vi "zad5.vi"() -> ()   [LabVIEW 2017]
panel:
  in  "Wybór podpunktu":enum32{"A", "B"}(radio)
  out "Suma":dbl
  in  "n":u64
  in  "r":dbl
  out "a(n)":dbl[](graph)
  in  "Wybierz ciąg":enum32{"Arytmetyczny", "Geometryczny"}(radio)
  in  "a1":dbl
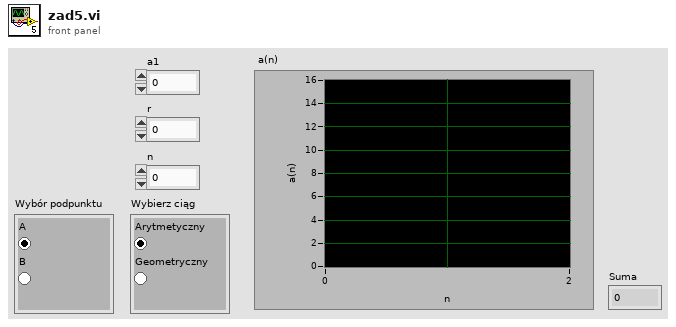
[diagram p1: front panel]
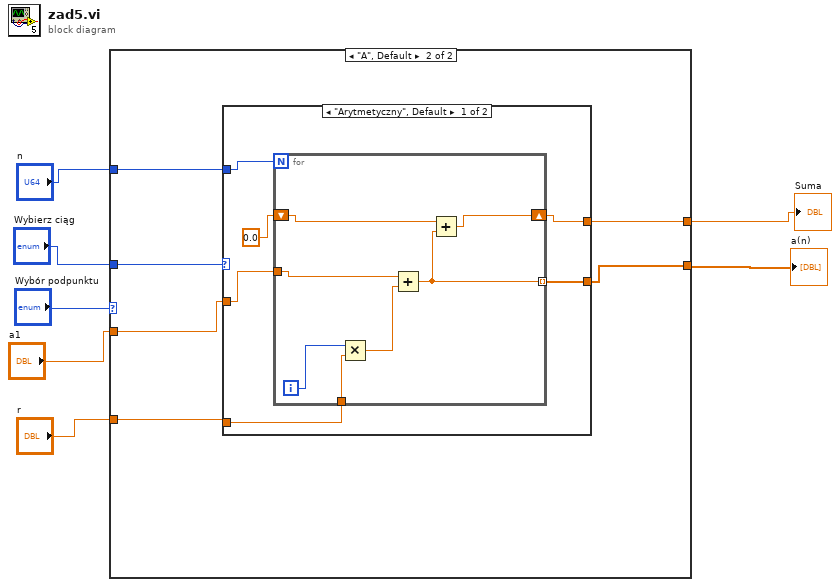
[diagram p0: block diagram]
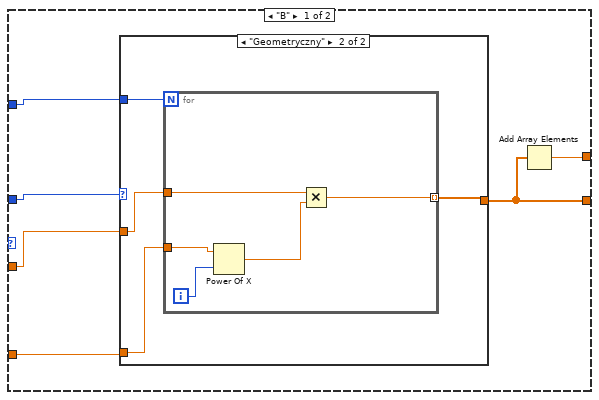
[diagram p2: hidden frame]
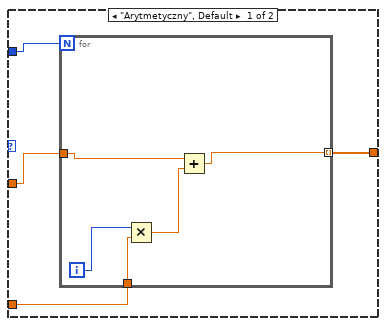
[diagram p3: hidden frame]
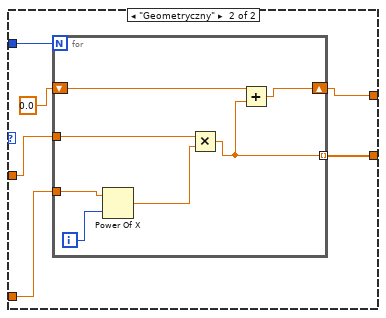
[diagram p4: hidden frame]
diagram:
  n1 = case shown="\"A\", Default" "Wybór podpunktu" {
    tunnel: [w8 w37] -> w2
    tunnel: "n" -> [w13 w36]
    tunnel: "r" -> [w10 w35]
    tunnel: "Wybierz ciąg" -> [w12 w34]
    tunnel: "a1" -> [w11 w33]
    tunnel: [w9 w32] -> w1
    frame "B" {
      n2 = case shown="\"Geometryczny\"" w12 {
        tunnel: w11 -> [w17 w25]
        tunnel: w10 -> [w16 w26]
        tunnel: w13 -> [w15 w24]
        tunnel: [w14 w23] -> w8
        frame "Arytmetyczny", Default {
          n3 = for {
            N: w15 -> [_]
            tunnel: w17 -> [w22]
            tunnel: w16 -> [w20]
            tunnel: [w18] -> w14 mode=indexing
            i -> [w21]
            n4 = Multiply(x=w21, y=w20) -> (x*y=w19:dbl)
            n5 = Add(x=w22, y=w19) -> (x+y=w18:dbl)
          }
        }
        frame "Geometryczny" {
          n6 = for {
            N: w24 -> [_]
            tunnel: w26 -> [w30]
            tunnel: w25 -> [w29]
            tunnel: [w27] -> w23 mode=indexing
            i -> [w31]
            n7 = Power Of X(1:w31, 2:w30) -> (0:w28:dbl)
            n8 = Multiply(x=w29, y=w28) -> (x*y=w27:dbl)
          }
        }
      }
      n9 = Add Array Elements(numeric array=w8) -> (sum=w9:dbl)
    }
    frame "A", Default {
      n10 = case shown="\"Arytmetyczny\", Default" w34 {
        tunnel: w33 -> [w43 w55]
        tunnel: w35 -> [w42 w56]
        tunnel: [w41 w54] -> w37
        tunnel: w36 -> [w40 w53]
        tunnel: [w38 w51] -> w32
        frame "Arytmetyczny", Default {
          n11 = for {
            N: w40 -> [_]
            tunnel: w43 -> [w50]
            tunnel: w42 -> [w48]
            tunnel: [w46] -> w41 mode=indexing
            shift-right: [w44] -> w38
            shift-left: 0.0 ("Numeric") -> [w45]
            i -> [w49]
            n12 = Multiply(x=w49, y=w48) -> (x*y=w47:dbl)
            n13 = Add(x=w50, y=w47) -> (x+y=w46:dbl)
            n14 = Add(x=w45, y=w46) -> (x+y=w44:dbl)
          }
        }
        frame "Geometryczny" {
          n15 = for {
            N: w53 -> [_]
            tunnel: w56 -> [w62]
            tunnel: w55 -> [w61]
            tunnel: [w59] -> w54 mode=indexing
            shift-right: [w57] -> w51
            shift-left: 0.0 ("Numeric") -> [w58]
            i -> [w63]
            n16 = Power Of X(1:w63, 2:w62) -> (0:w60:dbl)
            n17 = Multiply(x=w61, y=w60) -> (x*y=w59:dbl)
            n18 = Add(x=w58, y=w59) -> (x+y=w57:dbl)
          }
        }
      }
    }
  }
  "a(n)" <- w2
  "Suma" <- w1
